vi "删除1D数组元素(I64).vi"(8 "error in (no error)":errorcluster caption="错误输入（无错误）", 10 "索引":i32[](array[numeric]), 11 "输入数组":i64[](array[numeric])) -> (0 "error out":errorcluster caption="错误输出", 2 "已删除元素":i64[](array[numeric]), 3 "剩余元素":i64[](array[numeric]))   [LabVIEW 2012]
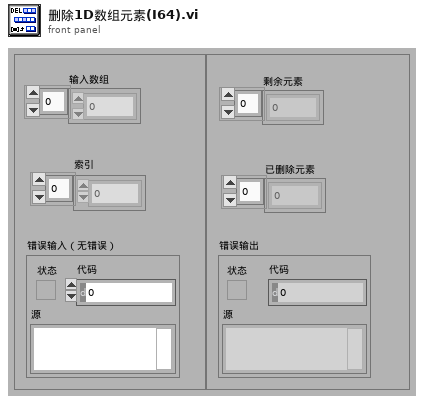
[diagram p1: front panel]
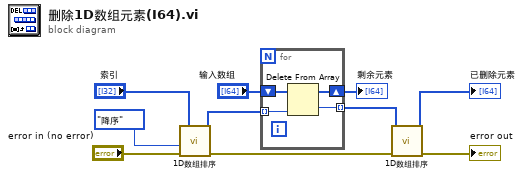
[diagram p0: block diagram]
diagram:
  n1 = call-poly "1D数组排序.vi"("error in (no error)"="error in (no error)", "升降序"=enum16{"升序", "降序"}."降序", "输入数组"="索引") -> ("error out"=w2:errorcluster, "排序后数组"=w6:i32[])  [unwired: 6 in, 1 out]
  n2 = for {
    shift-right: [w13] -> w4
    shift-left: "输入数组" -> [w14]
    tunnel: w6 -> [w12] mode=indexing
    tunnel: [w11] -> w5 mode=indexing
    n3 = Delete From Array(array=w14, index=w12) -> (deleted portion=w11:i64, array with subset deleted=w13:i64[])  [unwired: 1 in]
  }
  "剩余元素" <- w4
  n4 = call-poly "1D数组排序.vi"("error in (no error)"=w2, "输入数组"=w5) -> ("error out"=→"error out":errorcluster, "排序后数组"=→"已删除元素":i64[])  [unwired: 7 in, 1 out]
